vi "GeneratorBiasCurrents (1).vi"(10 "CurrentWaveForm":T1={"StartCurrent (mA)"=1.0, "MaximumCurrent (mA)"=3.0, "NumberOfCurrentPoints"=3, "NumberOfPointsInPulse"=20, "NumOfPointsAtPulseMAX"=4, "Exponent"=1} {"StartCurrent (mA)" min=0.001}) -> (0 "PulsedCurrentWaveForm":dbl[](array[numeric])=[0.0, 0.0, 0.0, 0.0, 0.0, 0.0, 0.0, 0.0, 0.0, 0.006819348298638839, 0.02709137914968268, 0.06026312439675552, 0.10542974530180321, 0.16135921418712945, 0.22652592093878654, 0.29915228767351526, 0.3772572564296004, 0.4587103272638338, 0.5412896727361661, 0.6227427435703996, 0.7008477123264847, 0.7734740790612133, 0.8386407858128705, 0.8945702546981968, 0.9397368756032445, 0.9729086208503173, 0.9931806517013612, 1.0, 1.0, 1.0, 1.0, 1.0, 1.0, 0.9931806517013612, 0.9729086208503173, 0.9397368756032445, 0.8945702546981968, 0.8386407858128706, 0.7734740790612135, 0.7008477123264847, 0.6227427435703996, 0.5412896727361662, 0.4587103272638339, 0.3772572564296004, 0.2991522876735153, 0.22652592093878665, 0.1613592141871295, 0.10542974530180316, 0.06026312439675552, 0.027091379149682737, 0.006819348298638839, 0.0, 0.0, 0.0, 0.0, 0.0, 0.0, 0.0, 0.0, 0.0, 0.0, 0.013638696597277677, 0.05418275829936536, 0.12052624879351104, 0.21085949060360643, 0.3227184283742589, 0.4530518418775731, 0.5983045753470305, 0.7545145128592008, 0.9174206545276676, 1.0825793454723323, 1.2454854871407992, 1.4016954246529694, 1.5469481581224267, 1.677281571625741, 1.7891405093963937, 1.879473751206489, 1.9458172417006345, 1.9863613034027223, 2.0, 2.0, 2.0, 2.0, 2.0, 2.0, 1.9863613034027223, 1.9458172417006345, 1.879473751206489, 1.7891405093963937, 1.6772815716257412, 1.546948158122427, 1.4016954246529694, 1.2454854871407992, 1.0825793454723325, 0.9174206545276677, 0.7545145128592008, 0.5983045753470306, 0.4530518418775733, 0.322718428374259, 0.21085949060360631, 0.12052624879351104, 0.054182758299365474, 0.013638696597277677, 0.0, 0.0, 0.0, 0.0, 0.0, 0.0, 0.0, 0.0, 0.0, 0.0, 0.020458044895916516, 0.08127413744904805, 0.18078937319026656, 0.31628923590540964, 0.48407764256138835, 0.6795777628163596, 0.8974568630205457, 1.1317717692888012, 1.3761309817915015, 1.6238690182084983, 1.8682282307111988, 2.1025431369794543, 2.32042223718364, 2.5159223574386114, 2.6837107640945908, 2.8192106268097334, 2.918725862550952, 2.9795419551040836, 3.0, 3.0, 3.0, 3.0, 3.0, 3.0, 2.9795419551040836, 2.918725862550952, 2.8192106268097334, 2.6837107640945903, 2.515922357438612, 2.3204222371836405, 2.1025431369794543, 1.8682282307111988, 1.6238690182084985, 1.3761309817915017, 1.1317717692888012, 0.8974568630205457, 0.67957776281636, 0.48407764256138863, 0.31628923590540925, 0.18078937319026656, 0.08127413744904821, 0.020458044895916405, 0.0], 2 "NumOfPointsAtPulseMIN":i32=8, 3 "CurrentStep (mA)":dbl=1.0)   [LabVIEW 2012]
panel:
  out "XY Graph":cluster{i32[], dbl[]}(graph)={[0, 1, 2, 3, 4, 5, 6, 7, 8, 9, 10, 11, 12, 13, 14, 15, 16, 17, 18, 19, 20, 21, 22, 23, 24, 25, 26, 27, 28, 29, 30, 31, 32, 33, 34, 35, 36, 37, 38, 39, 40, 41, 42, 43, 44, 45, 46, 47, 48, 49, 50, 51, 52, 53, 54, 55, 56, 57, 58, 59, 60, 61, 62, 63, 64, 65, 66, 67, 68, 69, 70, 71, 72, 73, 74, 75, 76, 77, 78, 79, 80, 81, 82, 83, 84, 85, 86, 87, 88, 89, 90, 91, 92, 93, 94, 95, 96, 97, 98, 99, 100, 101, 102, 103, 104, 105, 106, 107, 108, 109, 110, 111, 112, 113, 114, 115, 116, 117, 118, 119, 120, 121, 122, 123, 124, 125, 126, 127, 128, 129, 130, 131, 132, 133, 134, 135, 136, 137, 138, 139, 140, 141, 142, 143, 144, 145, 146, 147, 148, 149, 150, 151, 152, 153, 154, 155], [0.0, 0.0, 0.0, 0.0, 0.0, 0.0, 0.0, 0.0, 0.0, 0.006819348298638839, 0.02709137914968268, 0.06026312439675552, 0.10542974530180321, 0.16135921418712945, 0.22652592093878654, 0.29915228767351526, 0.3772572564296004, 0.4587103272638338, 0.5412896727361661, 0.6227427435703996, 0.7008477123264847, 0.7734740790612133, 0.8386407858128705, 0.8945702546981968, 0.9397368756032445, 0.9729086208503173, 0.9931806517013612, 1.0, 1.0, 1.0, 1.0, 1.0, 1.0, 0.9931806517013612, 0.9729086208503173, 0.9397368756032445, 0.8945702546981968, 0.8386407858128706, 0.7734740790612135, 0.7008477123264847, 0.6227427435703996, 0.5412896727361662, 0.4587103272638339, 0.3772572564296004, 0.2991522876735153, 0.22652592093878665, 0.1613592141871295, 0.10542974530180316, 0.06026312439675552, 0.027091379149682737, 0.006819348298638839, 0.0, 0.0, 0.0, 0.0, 0.0, 0.0, 0.0, 0.0, 0.0, 0.0, 0.013638696597277677, 0.05418275829936536, 0.12052624879351104, 0.21085949060360643, 0.3227184283742589, 0.4530518418775731, 0.5983045753470305, 0.7545145128592008, 0.9174206545276676, 1.0825793454723323, 1.2454854871407992, 1.4016954246529694, 1.5469481581224267, 1.677281571625741, 1.7891405093963937, 1.879473751206489, 1.9458172417006345, 1.9863613034027223, 2.0, 2.0, 2.0, 2.0, 2.0, 2.0, 1.9863613034027223, 1.9458172417006345, 1.879473751206489, 1.7891405093963937, 1.6772815716257412, 1.546948158122427, 1.4016954246529694, 1.2454854871407992, 1.0825793454723325, 0.9174206545276677, 0.7545145128592008, 0.5983045753470306, 0.4530518418775733, 0.322718428374259, 0.21085949060360631, 0.12052624879351104, 0.054182758299365474, 0.013638696597277677, 0.0, 0.0, 0.0, 0.0, 0.0, 0.0, 0.0, 0.0, 0.0, 0.0, 0.020458044895916516, 0.08127413744904805, 0.18078937319026656, 0.31628923590540964, 0.48407764256138835, 0.6795777628163596, 0.8974568630205457, 1.1317717692888012, 1.3761309817915015, 1.6238690182084983, 1.8682282307111988, 2.1025431369794543, 2.32042223718364, 2.5159223574386114, 2.6837107640945908, 2.8192106268097334, 2.918725862550952, 2.9795419551040836, 3.0, 3.0, 3.0, 3.0, 3.0, 3.0, 2.9795419551040836, 2.918725862550952, 2.8192106268097334, 2.6837107640945903, 2.515922357438612, 2.3204222371836405, 2.1025431369794543, 1.8682282307111988, 1.6238690182084985, 1.3761309817915017, 1.1317717692888012, 0.8974568630205457, 0.67957776281636, 0.48407764256138863, 0.31628923590540925, 0.18078937319026656, 0.08127413744904821, 0.020458044895916405, 0.0]}
  # "NumOfPointsAtPulseMax*2^(Exponent)=NumOfPointsAtPulseMIN"
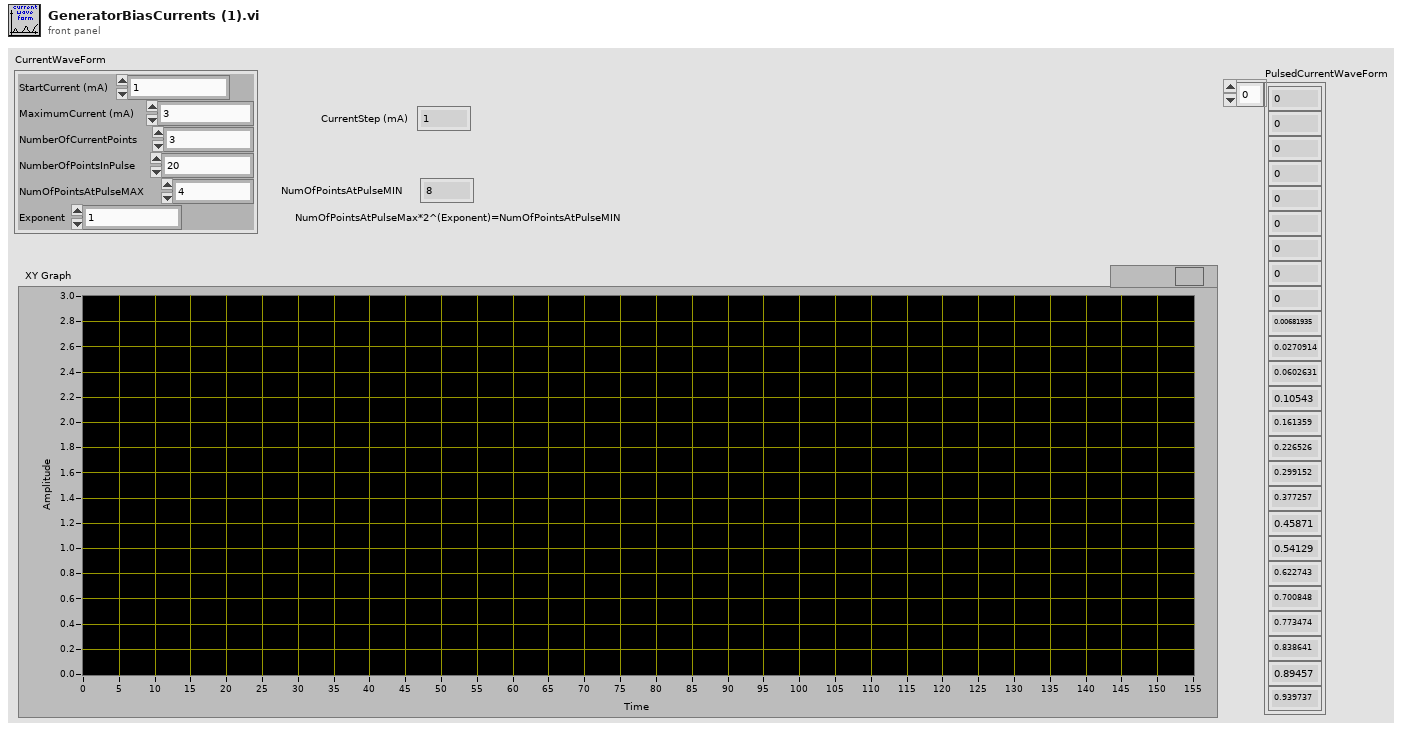
[diagram p1: front panel]
types:
  T1 = cluster{"StartCurrent (mA)":dbl, "MaximumCurrent (mA)":dbl, "NumberOfCurrentPoints":i32, "NumberOfPointsInPulse":i32, "NumOfPointsAtPulseMAX":i32, "Exponent":i16}
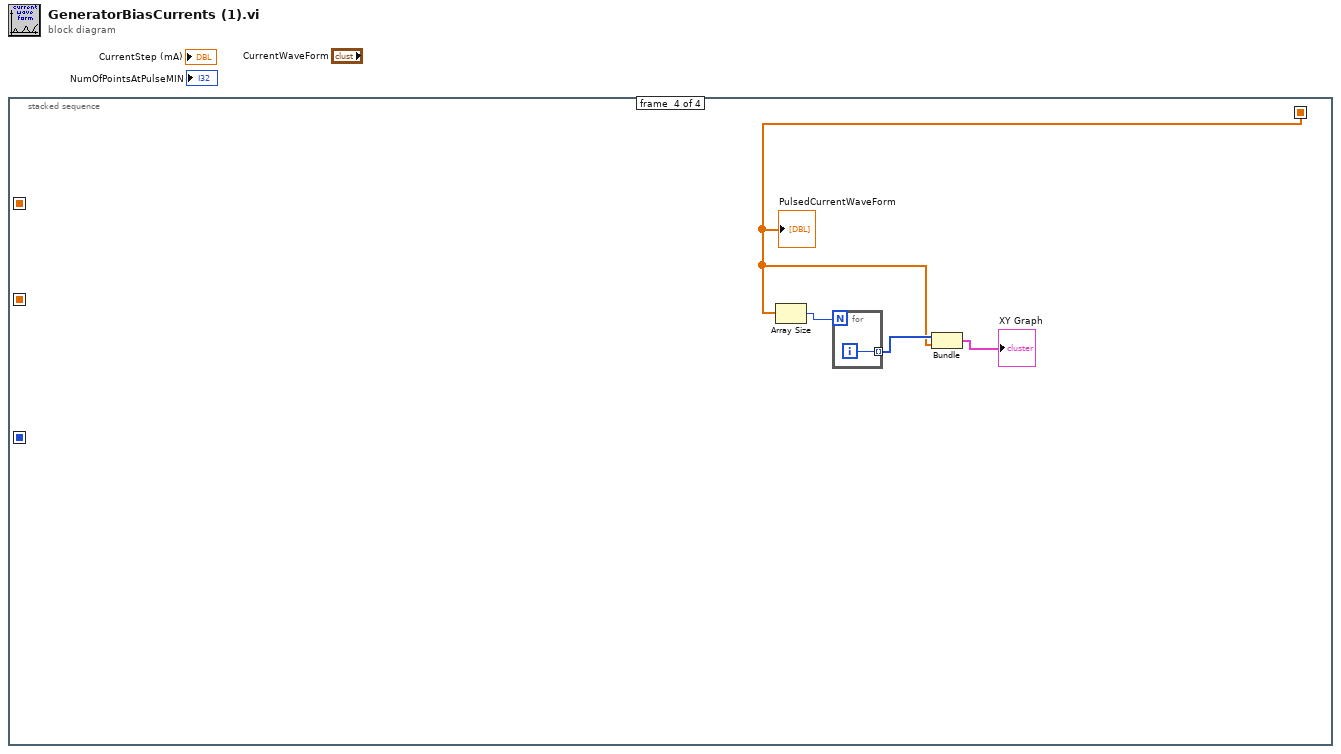
[diagram p0: block diagram]
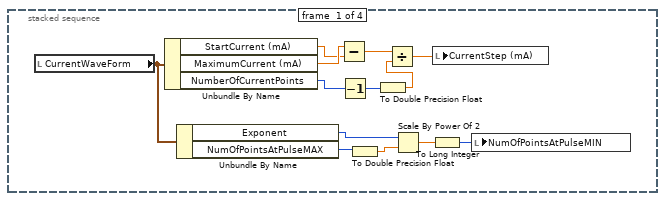
[diagram p2: hidden frame]
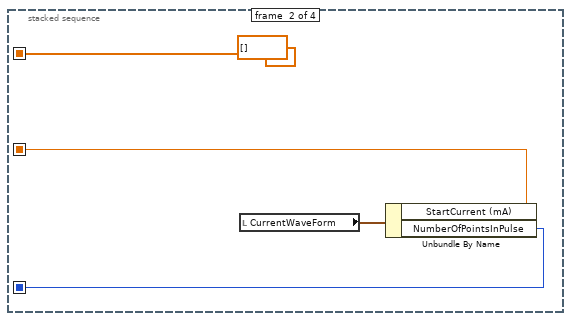
[diagram p3: hidden frame]
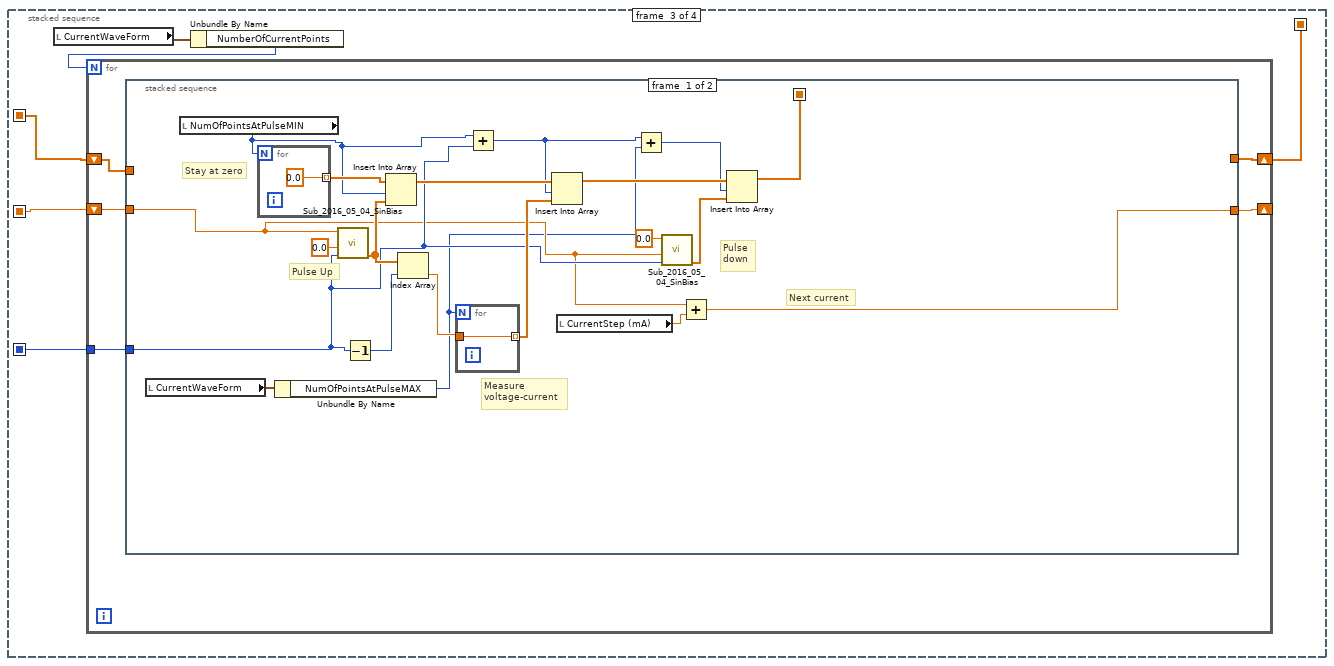
[diagram p4: hidden frame]
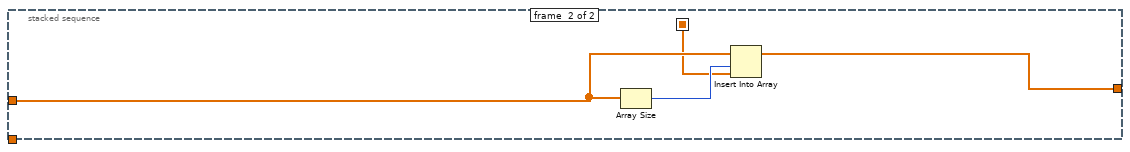
[diagram p5: hidden frame]
diagram:
  n1 = stacked-sequence {
    seq-local: [_ w16 _ _] -> [_ _ w21 _]
    seq-local: [_ w15 _ _] -> [_ _ w20 _]
    seq-local: [_ dbl[] [] _ _] -> [_ _ w19 _]
    seq-local: [_ _ w18 _] -> [_ _ _ w56]
    frame #0 {
      n2 = local read "CurrentWaveForm"() -> (w8:T1)
      n3 = Unbundle By Name(w8) -> ("StartCurrent (mA)"=w12:dbl, "MaximumCurrent (mA)"=w13:dbl, "NumberOfCurrentPoints"=w9:i32)
      n4 = Unbundle By Name(w8) -> ("Exponent"=w7:i16, "NumOfPointsAtPulseMAX"=w6:i32)
      n5 = Subtract(x=w13, y=w12) -> (x-y=w11:dbl)
      n6 = Decrement(x=w9) -> (x-1=w2:i32)
      n7 = To Double Precision Float(number=w6) -> (double precision float=w5:dbl)
      n8 = To Double Precision Float(number=w2) -> (double precision float=w1:dbl)
      n9 = Divide(x=w11, y=w1) -> (x/y=w10:dbl)
      n10 = Scale By Power Of 2(n=w7, x=w5) -> (x*2^n=w4:dbl)
      n11 = To Long Integer(number=w4) -> (32bit integer=w3:i32)
      n12 = local write "CurrentStep (mA)"(w10) -> ()
      n13 = local write "NumOfPointsAtPulseMIN"(w3) -> ()
    }
    frame #1 {
      n14 = local read "CurrentWaveForm"() -> (w17:T1)
      n15 = Unbundle By Name(w17) -> ("StartCurrent (mA)"=w16:dbl, "NumberOfPointsInPulse"=w15:i32)
    }
    frame #2 {
      n16 = local read "CurrentWaveForm"() -> (w23:T1)
      n17 = Unbundle By Name(w23) -> ("NumberOfCurrentPoints"=w22:i32)
      n18 = for {
        N: w22 -> [_]
        shift-right: [w26] -> _
        shift-left: w21 -> [w28]
        tunnel: w20 -> [w27]
        shift-right: [w24] -> w18
        shift-left: w19 -> [w25]
        n19 = stacked-sequence {
          seq-local: [w30 _] -> [_ w52]
          tunnel: w28 -> [w33 _]
          tunnel: w27 -> [w35 _]
          tunnel: [w31 _] -> w26
          tunnel: w25 -> [_ w54]
          tunnel: [_ w51] -> w24
          frame #0 {
            # "Stay at zero"
            # "Pulse Up"
            # "Pulse \ndown"
            # "Measure\nvoltage-current"
            # "Next current"
            n20 = local read "CurrentWaveForm"() -> (w41:T1)
            n21 = local read "NumOfPointsAtPulseMIN"() -> (w40:i32)
            n22 = for {
              N: w40 -> [_]
              tunnel: [0.0] -> w47 mode=indexing
            }
            n23 = Unbundle By Name(w41) -> ("NumOfPointsAtPulseMAX"=w29:i32)
            n24 = call "Sub_2016_05_04_SinBias.vi"("Number of steps"=w35, "Start current"=0.0, "Finish current"=w33) -> ("Array 2"=w46:dbl[])  [unwired: 7 in, 1 out]
            n25 = Decrement(x=w35) -> (x-1=w45:i32)
            n26 = Insert Into Array(array=w47, index=w40, new element=w46) -> (w43:dbl[])
            n27 = Index Array(array=w46, index=w45) -> (element=w44:dbl)
            n28 = for {
              N: w29 -> [_]
              tunnel: w44 -> [w49]
              tunnel: [w49] -> w42 mode=indexing
            }
            n29 = Add(x=w40, y=w35) -> (x+y=w36:i32)
            n30 = Insert Into Array(array=w43, index=w36, new element=w42) -> (w38:dbl[])
            n31 = local read "CurrentStep (mA)"() -> (w32:dbl)
            n32 = Add(x=w36, y=w29) -> (x+y=w34:i32)
            n33 = call "Sub_2016_05_04_SinBias.vi"("Number of steps"=w35, "Start current"=w33, "Finish current"=0.0) -> ("Array 2"=w37:dbl[])  [unwired: 7 in, 1 out]
            n34 = Add(x=w33, y=w32) -> (x+y=w31:dbl)
            n35 = Insert Into Array(array=w38, index=w34, new element=w37) -> (w30:dbl[])
          }
          frame #1 {
            n36 = Array Size(array=w54) -> (size(s)=w53:i32)
            n37 = Insert Into Array(array=w54, index=w53, new element=w52) -> (w51:dbl[])
          }
        }
      }
    }
    frame #3 {
      n38 = Array Size(array=w56) -> (size(s)=w58:i32)
      n39 = for {
        N: w58 -> [_]
        tunnel: [w59] -> w57 mode=indexing
        i -> [w59]
      }
      n40 = Bundle(w57, w56) -> (→"XY Graph":cluster{i32[], dbl[]})  [unwired: 1 in]
      "PulsedCurrentWaveForm" <- w56
    }
  }
